vi "Read CTR Channels.vi"(8 "error in (no error)":errorcluster, 11 "Task in":refnum<k21>) -> (0 "error out":errorcluster, 2 "1-Sample Waveforms":waveform(dbl)[](array[waveform]), 3 "Task out":refnum<k21>)   [LabVIEW 2021, in "Load Frame.lvlib"]
uses:
  Load Frame.lvlib
  <vilib>/DAQmx/read.llb/DAQmx Read (Counter DBL 1Chan 1Samp).vi
  <vilib>/DAQmx/miscellaneous.llb/DAQmx Fill In Error Info.vi
  Interval Timer/Interval Timer.lvlib
  <resource>/objmgr/daqmx.rc
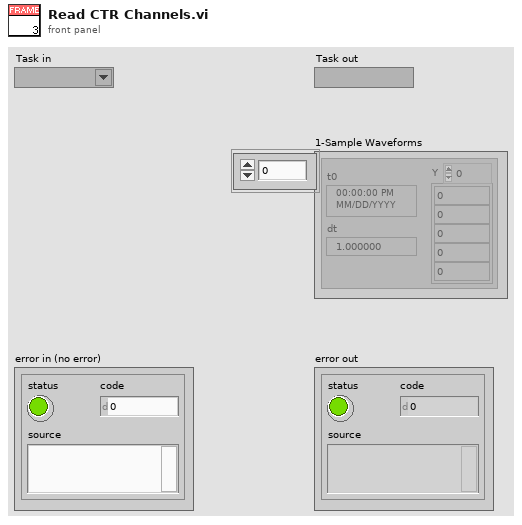
[diagram p1: front panel]
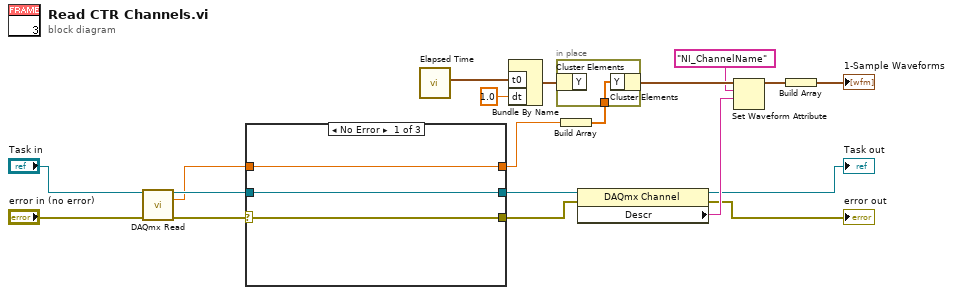
[diagram p0: block diagram]
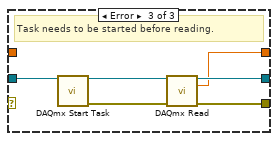
[diagram p3: hidden frame]
diagram:
  n1 = call-poly <vilib>:"DAQmx Read.vi"("task/channels in"="Task in", "error in"="error in (no error)") -> ("task out"=w9:refnum<k21>, "data"=w3:dbl, "error out"=w4:errorcluster)  [unwired: 11 in]
  n2 = case shown="No Error" w4 {
    selector: w4 -> [w21 w24 _]
    tunnel: w9 -> [w20 w23 w31]
    tunnel: [w20 w23 w29] -> w5
    tunnel: w3 -> [w22 w25 _]
    tunnel: [w22 w25 w26] -> w2
    tunnel: [w21 w24 w28] -> w1
    frame No Error {
    }
    frame Default {
      # "Propagate unknown errors."
    }
    frame Error {
      # "Task needs to be started before reading."
      n3 = call <vilib>:"DAQmx Start Task.vi"("task/channels in"=w31) -> ("task out"=w30:refnum<k21>, "error out"=w27:errorcluster)  [unwired: 13 in]
      n4 = call-poly <vilib>:"DAQmx Read.vi"("task/channels in"=w30, "error in"=w27) -> ("task out"=w29:refnum<k21>, "data"=w26:dbl, "error out"=w28:errorcluster)  [unwired: 11 in]
    }
  }
  n5 = call "Elapsed Time.vi"() -> ("current time"=w14:timestamp)  [unwired: 9 in, 2 out]
  n6 = Bundle By Name("t0"=w14, "dt"=1.0) -> (w16:waveform(dbl))  [unwired: 1 in]
  n7 = Build Array(w2) -> (w17:dbl[])
  n8 = in-place {
    in-place-border: w17 -> [w32]
    n9 = in-place-cluster #1(w16) -> ()  [unwired: 1 out]
    n10 = in-place-cluster #1("Y"=w32) -> (w19:waveform(dbl))
  }
  n11 = property class="DAQmx Channel"(reference=w5, error in=w1) -> (reference out=→"Task out":refnum<k21>, error out=→"error out":errorcluster, "Descr"=w8:string)
  n12 = Set Waveform Attribute(5:w8, 6:"NI_ChannelName" ("name"), 7:w19) -> (3:w11:waveform(dbl))  [unwired: 1 in, 2 out]
  n13 = Build Array(w11) -> (→"1-Sample Waveforms":waveform(dbl)[])
